vi "Write Channel Data.vi"(8 "error in (no error)":errorcluster, 10 "Channel Data":T1, 11 "Adc Convertor in":refnum<class "Adc Convertor.lvclass">) -> (0 "error out":errorcluster, 3 "Adc Convertor out":refnum<class "Adc Convertor.lvclass">)   [LabVIEW 2021, in "Adc Convertor.lvclass"]
uses:
  Adc Convertor.lvclass
  Controls/Channel Data.ctl
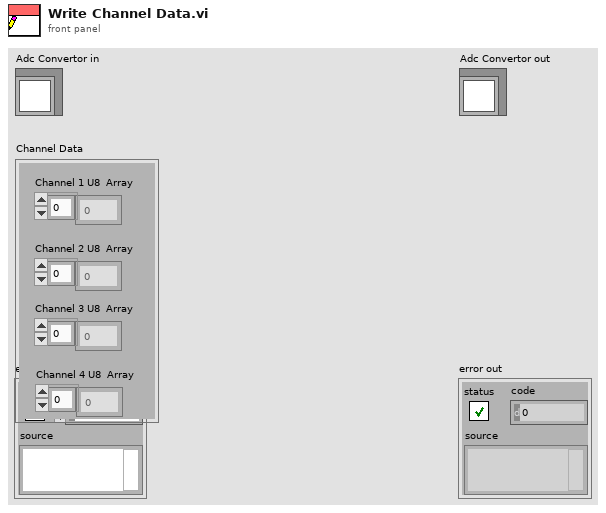
[diagram p1: front panel]
types:
  T1 = typedef "Channel Data.ctl" = cluster{"Channel 1 U8  Array":u8[], "Channel 2 U8  Array ":u8[], "Channel 3 U8  Array":u8[], "Channel 4 U8  Array":u8[]}
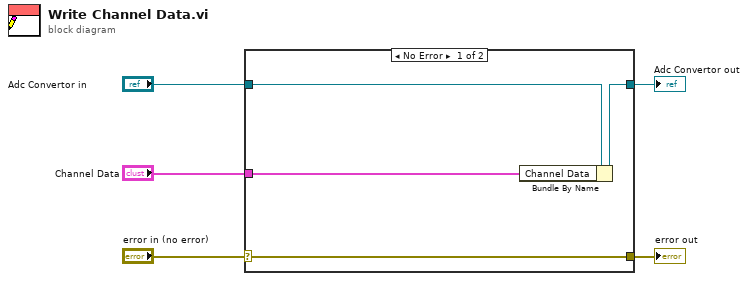
[diagram p0: block diagram]
diagram:
  n1 = case shown="No Error" "error in (no error)" {
    selector: "error in (no error)" -> [w9 w10]
    tunnel: [w9 w10] -> w4
    tunnel: [w7 w11] -> w2
    tunnel: "Adc Convertor in" -> [w8 w11]
    tunnel: "Channel Data" -> [w6 _]
    frame No Error {
      n2 = Bundle By Name(cluster=w8, "Channel Data"=w6) -> (w7:refnum<class "Adc Convertor.lvclass">)
    }
    frame Error {
    }
  }
  "error out" <- w4
  "Adc Convertor out" <- w2
